vi "MeasureSequenceSerialize.vi"(8 "error in":errorcluster, 9 "OwningElement in":refnum<k20>, 10 "Document in":refnum<k20>, 11 "Measure in":refnum<class "Measure.lvclass">) -> (0 "error out":errorcluster, 1 "OwningElement out":refnum<k20>, 2 "Document out":refnum<k20>, 3 "Measure out":refnum<class "Measure.lvclass">)   [LabVIEW 2021, in "ProligentXMLGenerator.lvlib" / "Measure.lvclass"]
uses:
  Measure.lvclass
  Measure.lvclass/Measure.ctl
  Model/Characteristic/Characteristic.lvclass
  Model/CustomData/CustomData.lvclass
  Failure/FailureReference/FailureReference.lvclass
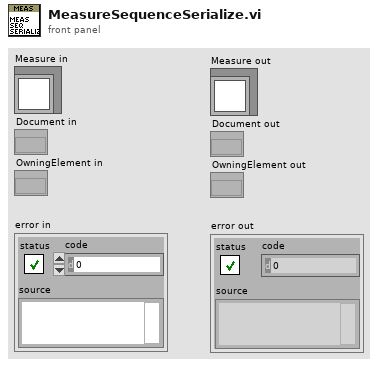
[diagram p1: front panel]
types:
  T1 = typedef "ProligentXMLGenerator.lvlib/Measure.lvclass/Data.ctl" = cluster{"Name":string, "Type":refnum<class "MeasureKind.lvclass">, "Precision":refnum<class "UnsignedByte.lvclass">, "Limit":refnum<class "MeasureLimit.lvclass">, "Characteristics":refnum<class "Characteristic.lvclass">[], "FailureReferences":refnum<class "FailureReference.lvclass">[], "CustomData":refnum<class "CustomData.lvclass">, "MeasureId":refnum<class "Guid.lvclass">, "MeasureTime":refnum<class "DateTime.lvclass">, "Comments":refnum<class "NonNullableString_TruncateAt_255.lvclass">, "Unit":refnum<class "NonEmptyString_30.lvclass">, "Symbol":refnum<class "NonEmptyString_20.lvclass">, "MeasureExecutionStatus":refnum<class "ExecutionStatus.lvclass">}
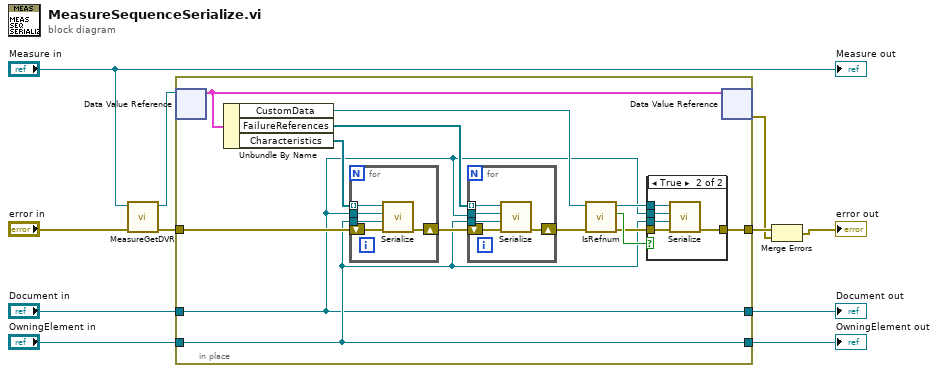
[diagram p0: block diagram]
diagram:
  n1 = call "MeasureGetDVR.vi"("error in"="error in", "Measure"="Measure in") -> ("error out"=w3:errorcluster, "DVRReference"=w2:refnum<data-value>)  [unwired: 8 in]
  n2 = in-place "In Place Element Structure" {
    in-place-border: [w23] -> w4
    in-place-border: "Document in" -> [w12]
    in-place-border: w3 -> [w19]
    in-place-border: "OwningElement in" -> [w13]
    in-place-border: [w13] -> w6
    in-place-border: [w12] -> w5
    n3 = in-place-dvr #1(w2) -> (w24:T1)  [unwired: 1 out]
    n4 = Unbundle By Name(w24) -> ("CustomData"=w20:refnum<class "CustomData.lvclass">, "FailureReferences"=w21:refnum<class "FailureReference.lvclass">[], "Characteristics"=w22:refnum<class "Characteristic.lvclass">[])
    n5 = for {
      tunnel: w22 -> [w34] mode=indexing
      tunnel: w13 -> [w32]
      tunnel: w12 -> [w33]
      shift-right: [w30] -> w15
      shift-left: w19 -> [w31]
      n6 = call "Serialize.vi"("error in"=w31, "OwningElement in"=w32, "Document in"=w33, "DocumentType in"=w34) -> ("error out"=w30:errorcluster)  [unwired: 4 in, 3 out]
    }
    n7 = for {
      tunnel: w21 -> [w29] mode=indexing
      tunnel: w13 -> [w27]
      tunnel: w12 -> [w28]
      shift-right: [w25] -> w14
      shift-left: w15 -> [w26]
      n8 = call "Serialize.vi"("error in"=w26, "OwningElement in"=w27, "Document in"=w28, "FailureReference in"=w29) -> ("error out"=w25:errorcluster)  [unwired: 4 in, 3 out]
    }
    n9 = call "IsRefnum.vi"("error in"=w14, "CustomDataType in"=w20) -> ("error out"=w16:errorcluster, "IsRefnum"=w18:bool, "CustomDataType out"=w17:refnum<class "CustomData.lvclass">)  [unwired: 7 in]
    n10 = case shown="True" w18 {
      tunnel: w12 -> [_ w37]
      tunnel: w16 -> [w35 w40]
      tunnel: [w35 w39] -> w23
      tunnel: w17 -> [_ w38]
      tunnel: w13 -> [_ w36]
      frame False {
      }
      frame True {
        n11 = call "Serialize.vi"("error in"=w40, "OwningElement in"=w36, "Document in"=w37, "CustomDataType in"=w38) -> ("error out"=w39:errorcluster)  [unwired: 4 in, 3 out]
      }
    }
    n12 = in-place-dvr #1(w24) -> (w1:errorcluster)  [unwired: 1 out]
  }
  "Document out" <- w5
  "OwningElement out" <- w6
  n13 = Merge Errors(w4, w1) -> (→"error out":errorcluster)
  "Measure out" <- "Measure in"
